vi "Publish to Endpoint.vi"(8 "error in (no error)":errorcluster, 9 "Message":string, 10 "Subject":string, 11 "Subscription in":refnum<class "Subscription.lvclass">) -> (0 "error out":errorcluster, 3 "Subscription out":refnum<class "Subscription.lvclass">)   [LabVIEW 2015, in "NI_AWS_SNS.lvlib" / "Subscription.lvclass"]
doc: "Sends a message to an Amazon SNS endpoint."
uses:
  Subscription.lvclass
  Core/HTTP Request/Request Options.ctl
  Core/HTTP Request/Name Value Pair.ctl
  Core/HTTP Request/Region handling.ctl
  Core/HTTP Request/URL formatting.ctl
  Subscription.lvclass/Subscription.ctl
  Read Topic.vi
  Core/HTTP Request/HTTP Request.lvclass
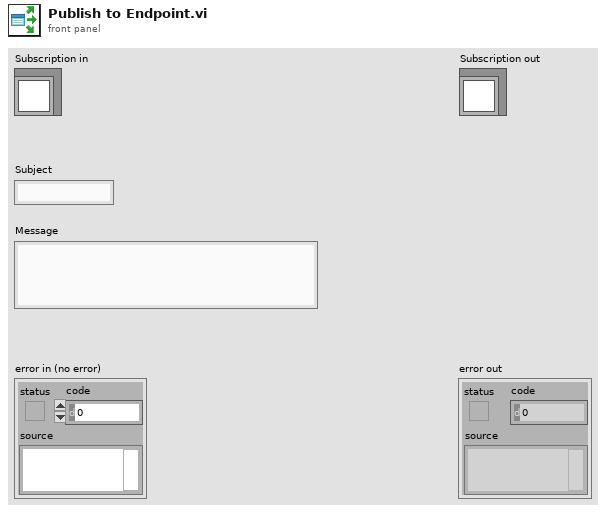
[diagram p1: front panel]
types:
  T1 = typedef "NI_AWS_Core.lvlib/HTTP Request.lvclass/Name Value Pair.ctl" = cluster{"name":string, "value":string}
  T2 = typedef "NI_AWS_Core.lvlib/HTTP Request.lvclass/Request Options.ctl" = cluster{"request headers":T1[], "request parameters":T1[], "request body":string, "region handling":T3, "URL formatting":T4}
  T3 = typedef "NI_AWS_Core.lvlib/HTTP Request.lvclass/Region handling.ctl" = enum16{"use region everywhere", "use region (authentication only)", "use region (URL only)", "ignore region everwhere"}
  T4 = typedef "NI_AWS_Core.lvlib/HTTP Request.lvclass/URL formatting.ctl" = enum16{"region-", "region."}
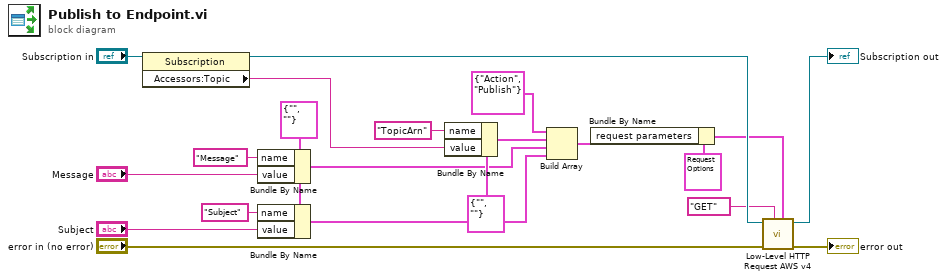
[diagram p0: block diagram]
diagram:
  w12 = T1 {"name"="", "value"=""} ("element")
  n1 = property class="Subscription"(reference="Subscription in") -> (reference out=w3:refnum<class "Subscription.lvclass">, "Accessors:Topic"=w15:string)  [unwired: 1 in, 1 out]
  n2 = Bundle By Name(cluster=w12, "name"="Message", "value"="Message") -> (w14:T1)
  n3 = Bundle By Name(cluster=w12, "name"="Subject", "value"="Subject") -> (w13:T1)
  n4 = Bundle By Name(cluster=T1 {"name"="", "value"=""} ("Name Value Pair"), "name"="TopicArn", "value"=w15) -> (w17:T1)
  n5 = Build Array(T1 {"name"="Action", "value"="Publish"} ("Name Value Pair"), w17, w14, w13) -> (w20:T1[])
  n6 = Bundle By Name(cluster=T2 {"request headers"=[], "request parameters"=[], "request body"="", "region handling"=enum."use region everywhere", "URL formatting"=enum."region."} ("Request Options"), "request parameters"=w20) -> (w2:T2)
  n7 = call "Low-Level HTTP Request AWS v4.vi"("Request Options"=w2, "HTTP-Verb"="GET", "error in (no error)"="error in (no error)", "AWS Core in"=w3) -> ("error out"=→"error out":errorcluster, "AWS Core out"=→"Subscription out":refnum<class "Subscription.lvclass">)  [unwired: 4 in, 2 out]
